vi "Controle_velocidade_servo (SubVI).vi"(7 "Channel Name":tag, 8 "error in (no error)":errorcluster, 9 "Posição Desejada":dbl, 10 "y":dbl, 11 "milliseconds to wait":u32) -> (0 "error out":errorcluster, 2 "Duty Cycle":dbl(slide)=1.5 scale=0.025..0.125, 3 "Posição":dbl(knob)=1.5 scale=0.0..200.0)   [LabVIEW 2017]
uses:
  <vilib>/myRIO/Common/Instrument Driver Framework/myRIO v1.0/PWM/vis/myRIO v1.0 Close PWM.vi
  <vilib>/myRIO/Common/Instrument Driver Framework/myRIO v1.0/PWM/vis/myRIO v1.0 Unreserve PWM.vi
  <vilib>/myRIO/Common/Instrument Driver Framework/myRIO v1.0/PWM/vis/myRIO v1.0 Build MUX Configuration PWM.vi
  <vilib>/myRIO/Common/Instrument Driver Framework/myRIO v1.0/Resource Manager/vis/myRIO v1.0 Unreserve Channel List.vi
  <vilib>/myRIO/Common/Instrument Driver Framework/myRIO v1.0/Resource Manager/vis/myRIO v1.0 Create Configuration List.vi
  <vilib>/myRIO/Common/Instrument Driver Framework/myRIO v1.0/Resource Manager/vis/myRIO v1.0 Unreserve Channel.vi
  <vilib>/myRIO/Common/Instrument Driver Framework/myRIO v1.0/Resource Manager/vis/myRIO v1.0 Build Mutex Name.vi
  <vilib>/Utility/error.llb/Error Cluster From Error Code.vi
  <vilib>/myRIO/Common/Instrument Driver Framework/myRIO v1.0/PWM/vis/myRIO v1.0 Write PWM.vi
  <vilib>/myRIO/Common/Instrument Driver Framework/myRIO v1.0/PWM/vis/myRIO v1.0 Shutdown PWM.vi
  <vilib>/myRIO/Common/Instrument Driver Framework/myRIO v1.0/Resource Manager/vis/myRIO v1.0 Configure IO.vi
  <vilib>/myRIO/Common/Instrument Driver Framework/Utilities/vis/Configuration Manager.vi
  <vilib>/myRIO/Common/Instrument Driver Framework/Utilities/vis/IO Manager.vi
  <vilib>/myRIO/Common/Instrument Driver Framework/myRIO v1.0/myRIO v1.0 Close.vi
  <vilib>/myRIO/Instrument Drivers/Onboard IO/PWM/PWM.lvlib
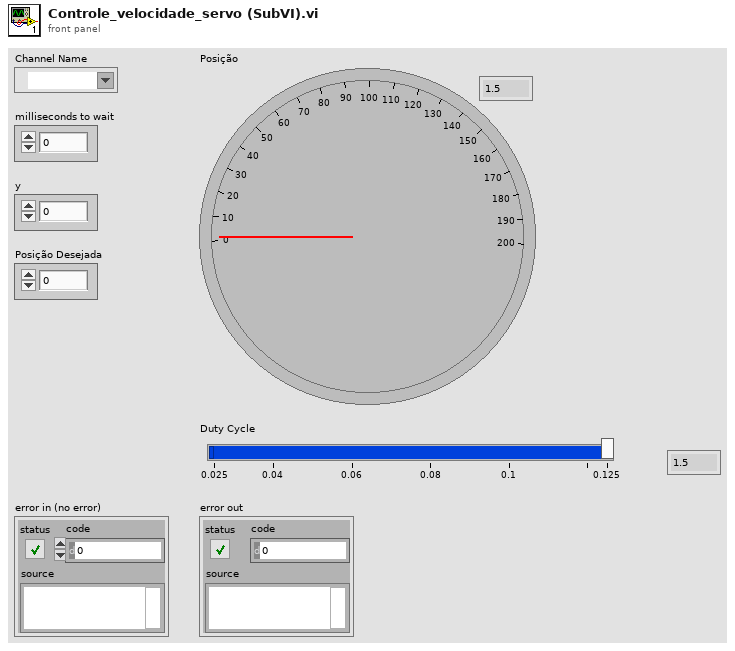
[diagram p1: front panel]
types:
  T1 = typedef "PWM.lvlib/PWM Reference.ctl" = cluster{"myRIO Reference":T2, "PWM Channels Enum":T6, "PWM Configuration":T7}
  T2 = typedef "myRIO Generic Hardware Reference.ctl" = cluster{"myRIO Model":T3, "myRIO Hardware Reference":T4}
  T3 = typedef "Hardware Version Enum.ctl" = enum16{"Unknown", "myRIO-1900", "myRIO-1950", "roboRIO", "NI ELVIS RIO CM"}
  T4 = typedef "myRIO v1.0 Reference.ctl" = cluster{"Generic FPGA Reference":T5, "Allow multiple opens":bool}
  T5 = typedef "Generic FPGA Reference.ctl" = refnum<k20>
  T6 = typedef "PWM Channels Enum.ctl" = enum16{"Not Connected", "C/PWM0", "C/PWM1", "A/PWM0", "A/PWM1", "A/PWM2", "B/PWM0", "B/PWM1", "B/PWM2", "PWM/PWM0", "PWM/PWM1", "PWM/PWM2", "PWM/PWM3", "PWM/PWM4", "PWM/PWM5", "PWM/PWM6", "PWM/PWM7", "PWM/PWM8", "PWM/PWM9"}
  T7 = typedef "PWM.lvlib/PWM Configuration.ctl" = cluster{"Frequency":dbl, "Duty Cycle":dbl}
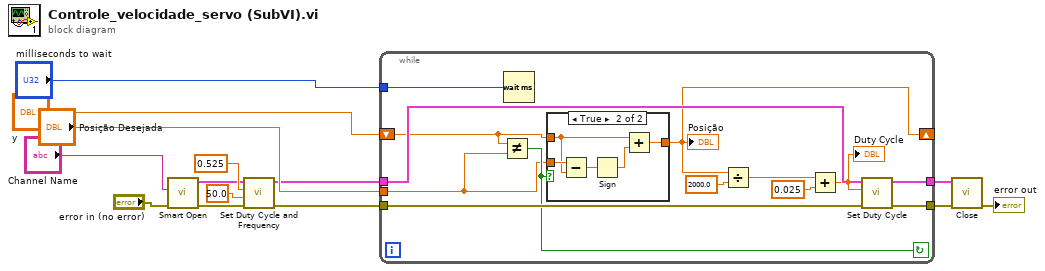
[diagram p0: block diagram]
diagram:
  n1 = call <vilib>:"Smart Open.vi"("error in (no error)"="error in (no error)", "Channel Name"="Channel Name") -> ("error out"=w4:errorcluster, "PWM Ref Out"=w5:T1)  [unwired: 8 in]
  n2 = call <vilib>:"Set Duty Cycle and Frequency.vi"("error in (no error)"=w4, "Frequency [Hz]"=50.0, "Duty Cycle"=0.525, "PWM Ref In"=w5) -> ("error out"=w8:errorcluster, "PWM Ref Out"=w7:T1)  [unwired: 5 in]
  n3 = while {
    tunnel: w7 -> [w26]
    tunnel: w8 -> [w27]
    tunnel: [w25] -> w11
    shift-right: [w19] -> _
    shift-left: "y" -> [w20]
    tunnel: [w18] -> w12
    tunnel: "milliseconds to wait" -> [w17]
    tunnel: "Posição Desejada" -> [w15]
    stop <- w16 continue-if-true
    n4 = Not Equal?(x=w20, y=w15) -> (x != y?=w16:bool)
    n5 = Wait (ms)(milliseconds to wait=w17) -> ()  [unwired: 1 out]
    n6 = case shown="True" w16 {
      tunnel: w15 -> [_ w33]
      tunnel: w20 -> [w28 w31]
      tunnel: [w28 w30] -> w19
      frame False {
      }
      frame True {
        n7 = Subtract(x=w33, y=w31) -> (x-y=w32:dbl)
        n8 = Sign(1:w32) -> (0:w29:dbl)
        n9 = Add(x=w31, y=w29) -> (x+y=w30:dbl)
      }
    }
    "Posição" <- w19
    n10 = Divide(x=w19, y=2000.0) -> (x/y=w23:dbl)
    n11 = Add(x=w23, y=0.025) -> (x+y=w21:dbl)
    "Duty Cycle" <- w21
    n12 = call <vilib>:"Set Duty Cycle.vi"("error in (no error)"=w27, "Duty Cycle"=w21, "PWM Ref In"=w26) -> ("error out"=w25:errorcluster, "PWM Ref Out"=w18:T1)  [unwired: 6 in]
  }
  n13 = call <vilib>:"Close.vi"("error in (no error)"=w11, "PWM Ref In"=w12) -> ("error out"=→"error out":errorcluster)  [unwired: 9 in]
